vi "CSM - Keywords.vi"() -> (2 "%[hex] Code":string[](array[string]), 3 "Source":string[](array[string]))   [LabVIEW 2020, in "Communicable State Machine.lvlib"]
uses:
  Communicable State Machine.lvlib
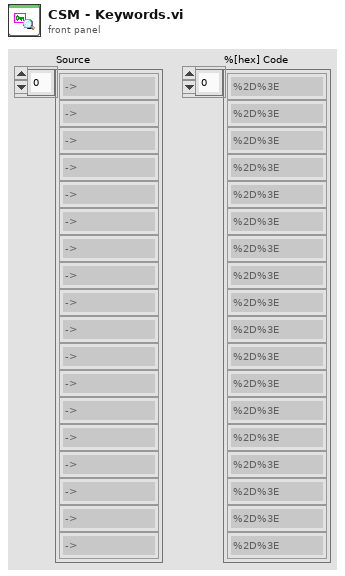
[diagram p1: front panel]
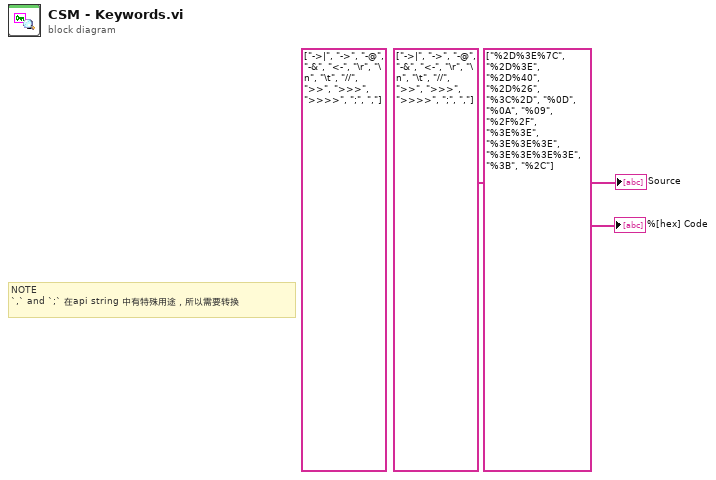
[diagram p0: block diagram]
diagram:
  (unwired) string[] ["->|", "->", "-@", "-&", "<-", "\r", "\n", "\t", "//", ">>", ">>>", ">>>>", ";", ","]
  # "NOTE\n`,` and `;` 在api string 中有特殊用途，所以需要转换"
  "%[hex] Code" <- string[] ["%2D%3E%7C", "%2D%3E", "%2D%40", "%2D%26", "%3C%2D", "%0D", "%0A", "%09", "%2F%2F", "%3E%3E", "%3E%3E%3E", "%3E%3E%3E%3E", "%3B", "%2C"]
  "Source" <- string[] ["->|", "->", "-@", "-&", "<-", "\r", "\n", "\t", "//", ">>", ">>>", ">>>>", ";", ","]
